vi "梦幻城堡C6~20通信.vi"() -> ()   [LabVIEW 2016, in "环境动力监测库.lvlib" / "UPS库.lvlib"]
uses:
  <vilib>/Instr/_visa.llb/VISA Configure Serial Port (Instr).vi
panel:
  out "Status-WA":T1
  out "Status-Q6":T2
  in  "open":bool
  in  "close":bool
  out "通信指示":bool
  in  "关机":bool
  in  "功率查询":bool
  in  "状态查询":bool
  out "读取缓冲区":string
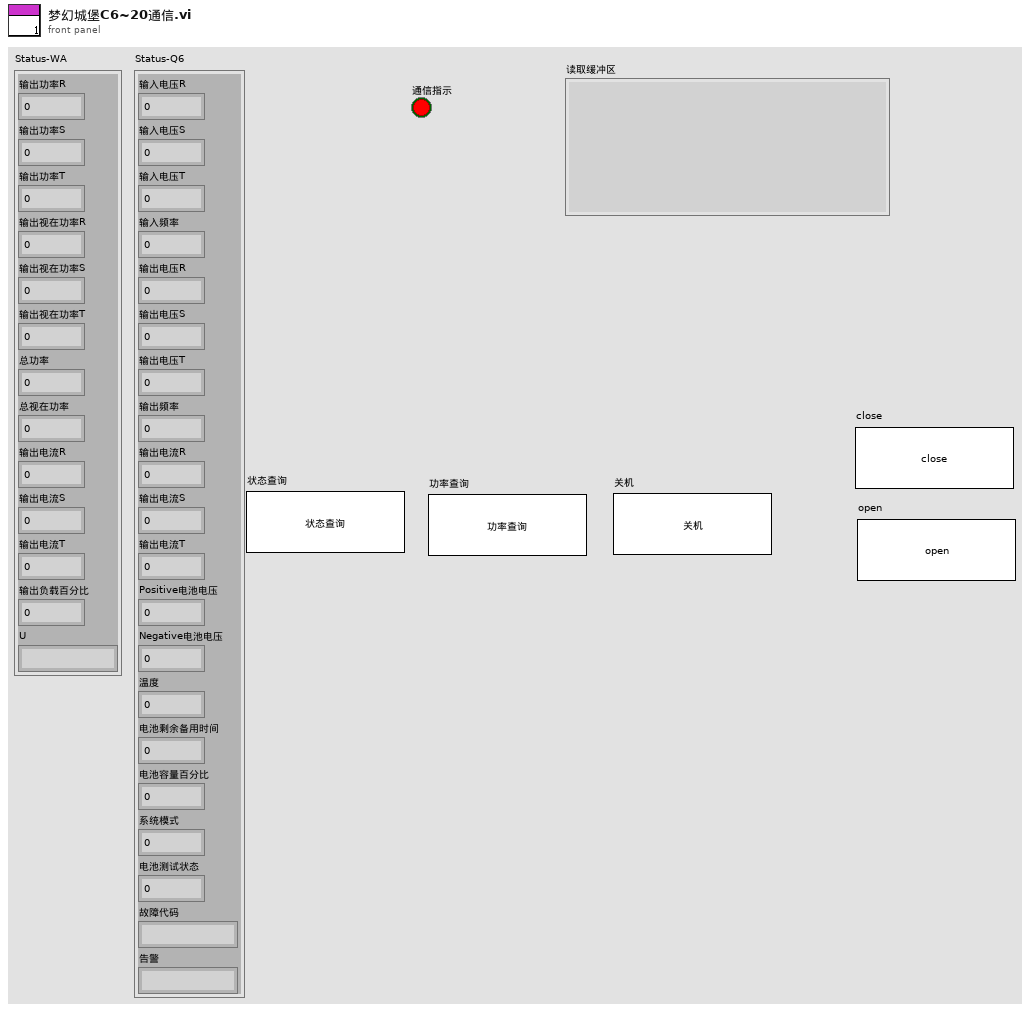
[diagram p1: front panel]
types:
  T1 = cluster{"输出功率R":dbl, "输出功率S":dbl, "输出功率T":dbl, "输出视在功率R":dbl, "输出视在功率S":dbl, "输出视在功率T":dbl, "总功率":dbl, "总视在功率":dbl, "输出电流R":dbl, "输出电流S":dbl, "输出电流T":dbl, "输出负载百分比":dbl, "U":string}
  T2 = cluster{"输入电压R":dbl, "输入电压S":dbl, "输入电压T":dbl, "输入频率":dbl, "输出电压R":dbl, "输出电压S":dbl, "输出电压T":dbl, "输出频率":dbl, "输出电流R":dbl, "输出电流S":dbl, "输出电流T":dbl, "Positive电池电压":dbl, "Negative电池电压":dbl, "温度":dbl, "电池剩余备用时间":dbl, "电池容量百分比":dbl, "系统模式":dbl, "电池测试状态":dbl, "故障代码":string, "告警":string}
  T3 = cluster{"枚举":enum16{"open", "read", "write", "close"}, "写入缓冲区":string}
  T4 = cluster{"VISA resource name":refnum<visa-resource-name>, "Serial Config":cluster{"baud rate (9600)":u32, "stop bits (10: 1 bit)":u16, "parity (0:none)":enum16{"None", "Odd", "Even", "Mark", "Space"}, "data bits (8)":u16, "timeout (10sec)":u32}, "型号选择":enum16{"山特UPSC1~3", "山特UPSC6~20", "华为UPS2000-G-(1-3KVA)"}, "HW-UPS-2000 MB session":refnum<class "MB_Master.lvclass">, "连接方式":enum16{"串口", "TCP"}, "IP":string, "Port":string}
  T5 = cluster{"baud rate (9600)":u32, "stop bits (10: 1 bit)":u16, "parity (0:none)":enum16{"None", "Odd", "Even", "Mark", "Space"}, "data bits (8)":u16, "timeout (10sec)":u32}
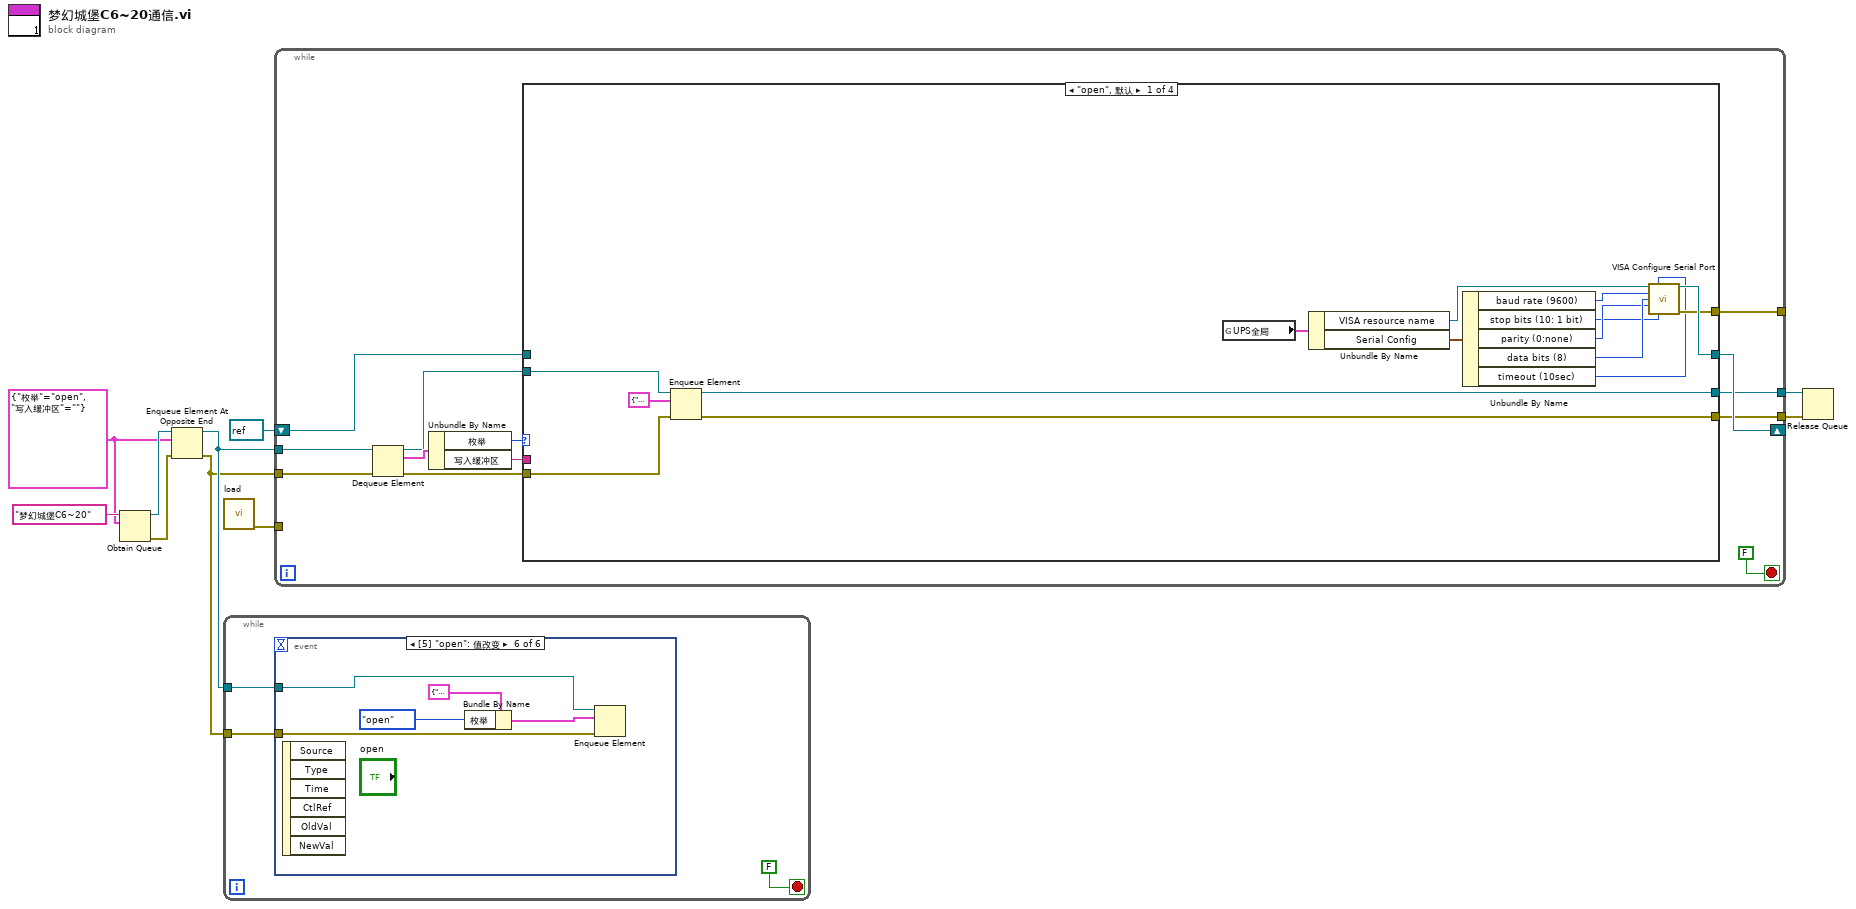
[diagram p0: block diagram]
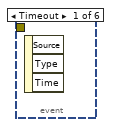
[diagram p2: hidden frame]
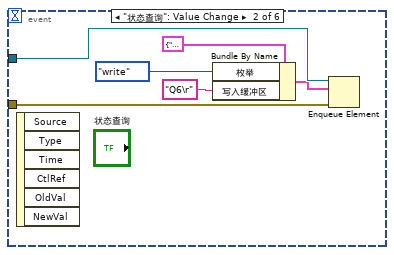
[diagram p3: hidden frame]
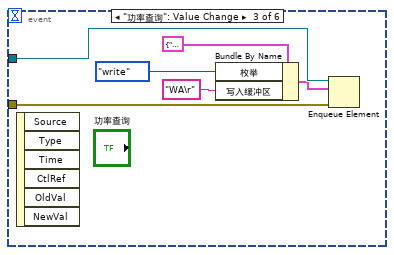
[diagram p4: hidden frame]
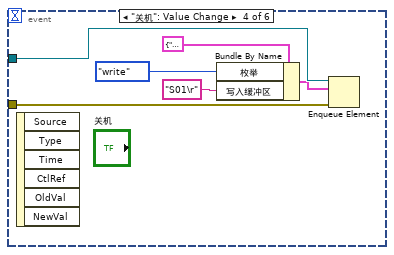
[diagram p5: hidden frame]
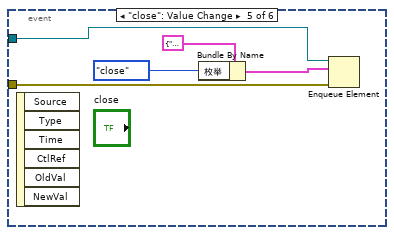
[diagram p6: hidden frame]
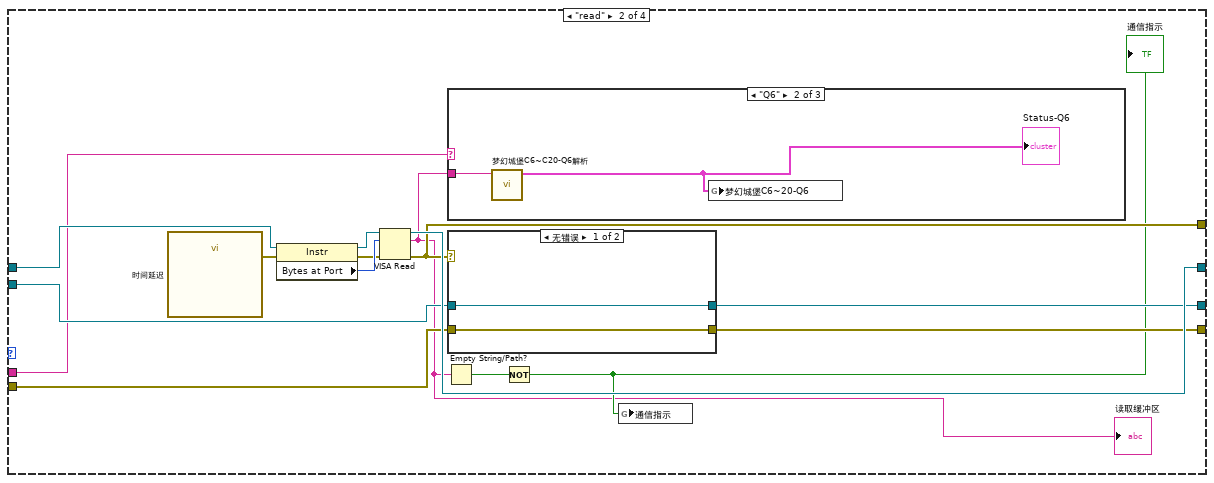
[diagram p7: hidden frame]
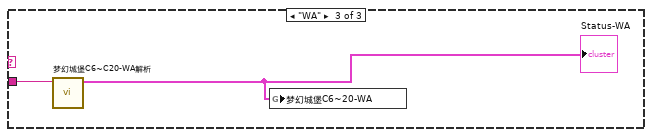
[diagram p9: hidden frame]
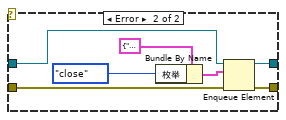
[diagram p10: hidden frame]
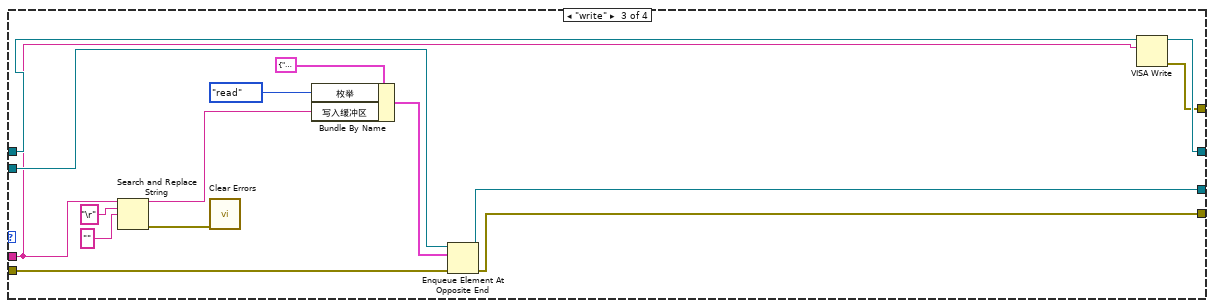
[diagram p11: hidden frame]
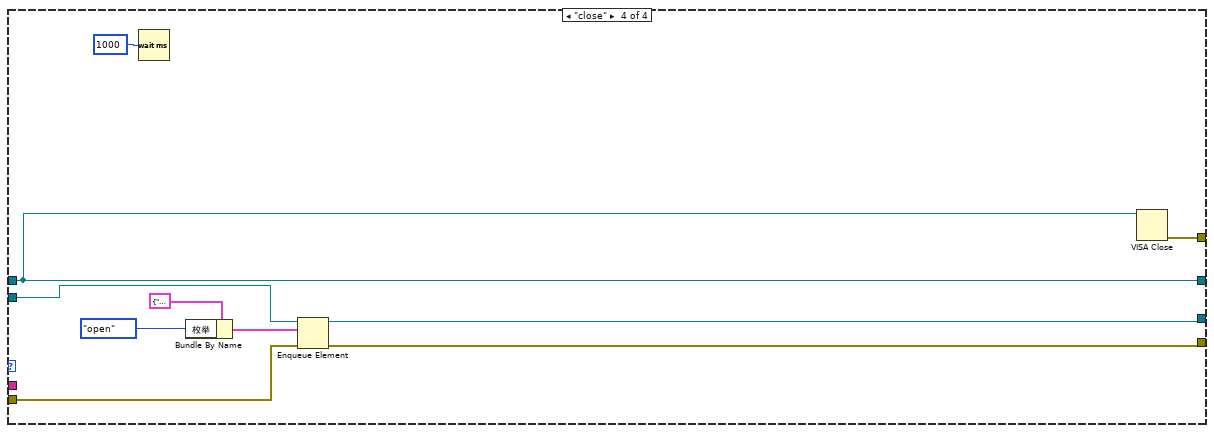
[diagram p12: hidden frame]
diagram:
  w5 = T3 {"枚举"=enum."open", "写入缓冲区"=""}
  n1 = Obtain Queue(name (unnamed)="梦幻城堡C6~20" ("名称（未命名）"), element data type=w5) -> (queue out=w9:refnum<queue>, error out=w8:errorcluster)  [unwired: 3 in, 1 out]
  n2 = Enqueue Element At Opposite End(queue=w9, element=w5, error in (no error)=w8) -> (queue out=w7:refnum<queue>, error out=w6:errorcluster)  [unwired: 1 in, 1 out]
  n3 = call "load.vi"() -> ("error out"=w1:errorcluster)  [unwired: 11 in]
  n4 = while {
    tunnel: w7 -> [w12]
    tunnel: w6 -> [w11]
    stop <- FALSE stop-if-true
    n5 = event shown="[5] \"open\": 值改变" {
      selector: _ -> [_ _ _ _ _ _]
      dyn-events: _ -> [_ _ _ _ _ _]
      timeout: _ -> [_ _ _ _ _ _]
      tunnel: w12 -> [_ w19 w25 w31 w36 w41]
      tunnel: w11 -> [_ w18 w24 w30 w35 w40]
      event Timeout {
        n6 = event-data() -> ()  [unwired: 1 in, 3 out]
      }
      event "状态查询": Value Change {
        n7 = event-data() -> ()  [unwired: 1 in, 6 out]
        n8 = Bundle By Name(cluster=T3 {"枚举"=enum."open", "写入缓冲区"=""}, "枚举"=enum16{"open", "read", "write", "close"}."write" ("元素"), "写入缓冲区"="Q6\r") -> (w14:T3)
        n9 = Enqueue Element(queue=w19, element=w14, error in (no error)=w18) -> ()  [unwired: 1 in, 3 out]
      }
      event "功率查询": Value Change {
        n10 = event-data() -> ()  [unwired: 1 in, 6 out]
        n11 = Bundle By Name(cluster=T3 {"枚举"=enum."open", "写入缓冲区"=""}, "枚举"=enum16{"open", "read", "write", "close"}."write" ("元素"), "写入缓冲区"="WA\r") -> (w20:T3)
        n12 = Enqueue Element(queue=w25, element=w20, error in (no error)=w24) -> ()  [unwired: 1 in, 3 out]
      }
      event "关机": Value Change {
        n13 = event-data() -> ()  [unwired: 1 in, 6 out]
        n14 = Bundle By Name(cluster=T3 {"枚举"=enum."open", "写入缓冲区"=""}, "枚举"=enum16{"open", "read", "write", "close"}."write" ("元素"), "写入缓冲区"="S01\r") -> (w26:T3)
        n15 = Enqueue Element(queue=w31, element=w26, error in (no error)=w30) -> ()  [unwired: 1 in, 3 out]
      }
      event "close": Value Change {
        n16 = event-data() -> ()  [unwired: 1 in, 6 out]
        n17 = Bundle By Name(cluster=T3 {"枚举"=enum."open", "写入缓冲区"=""}, "枚举"=enum16{"open", "read", "write", "close"}."close") -> (w32:T3)
        n18 = Enqueue Element(queue=w36, element=w32, error in (no error)=w35) -> ()  [unwired: 1 in, 3 out]
      }
      event "open": Value Change {
        n19 = event-data() -> ()  [unwired: 1 in, 6 out]
        n20 = Bundle By Name(cluster=T3 {"枚举"=enum."open", "写入缓冲区"=""}, "枚举"=enum16{"open", "read", "write", "close"}."open") -> (w37:T3)
        n21 = Enqueue Element(queue=w41, element=w37, error in (no error)=w40) -> ()  [unwired: 1 in, 3 out]
      }
    }
  }
  n22 = while {
    shift-right: [w54] -> _
    shift-left: refnum<visa-resource-name> refnum ("VISA resource name out") -> [w53]
    tunnel: [w52] -> _
    tunnel: w7 -> [w50]
    tunnel: w6 -> [w49]
    tunnel: [w44] -> w3
    tunnel: [w43] -> w2
    tunnel: w1 -> [_]
    stop <- FALSE stop-if-true
    n23 = Dequeue Element(queue=w50, error in (no error)=w49) -> (queue out=w46:refnum<queue>, element=w48:T3, error out=w45:errorcluster)  [unwired: 1 in, 1 out]
    n24 = Unbundle By Name(w48) -> ("枚举"=w47:enum16{"open", "read", "write", "close"}, "写入缓冲区"=w42:string)
    n25 = case shown="\"open\", 默认" w47 {
      tunnel: [w69 w81 w111 w121] -> w54
      tunnel: w53 -> [_ w84 w112 w121]
      tunnel: [w68 w79 w110 w122] -> w52
      tunnel: w46 -> [w61 w78 w103 w117]
      tunnel: w45 -> [w60 w77 w102 w116]
      tunnel: [w59 w76 w101 w115] -> w44
      tunnel: [w58 w75 w100 w114] -> w43
      tunnel: w42 -> [_ w74 w98 _]
      frame "open", Default {
        n26 = Enqueue Element(queue=w61, element=T3 {"枚举"=enum."read", "写入缓冲区"=""}, error in (no error)=w60) -> (queue out=w59:refnum<queue>, error out=w58:errorcluster)  [unwired: 1 in, 1 out]
        n27 = global read "断电保存全局变量.vi" "UPS全局"() -> (w57:T4)
        n28 = Unbundle By Name(w57) -> ("VISA resource name"=w55:refnum<visa-resource-name>, "Serial Config"=w56:T5)
        n29 = Unbundle By Name(w56) -> ("baud rate (9600)"=w66:u32, "stop bits (10: 1 bit)"=w63:u16, "parity (0:none)"=w64:enum16{"None", "Odd", "Even", "Mark", "Space"}, "data bits (8)"=w65:u16, "timeout (10sec)"=w67:u32)
        n30 = call-poly "VISA Configure Serial Port"("VISA resource name"=w55, "timeout (10sec)"=w67, "baud rate (9600)"=w66, "data bits (8)"=w65, "parity (0:none)"=w64, "stop bits (10: 1 bit)"=w63) -> ("VISA resource name out"=w69:refnum<visa-resource-name>, "error out"=w68:errorcluster)  [unwired: 8 in]
      }
      frame "read" {
        n31 = call "时间延迟"() -> ("error out"=w80:errorcluster)  [unwired: 11 in]
        n32 = property class="Instr"(reference=w84, error in=w80) -> (reference out=w82:refnum<visa-resource-name>, error out=w73:errorcluster, "Bytes at Port"=w83:u32)
        n33 = VISA Read(VISA resource name=w82, byte count=w83, error in (no error)=w73) -> (VISA resource name out=w81:refnum<visa-resource-name>, read buffer=w71:string, error out=w79:errorcluster)  [unwired: 1 out]
        "读取缓冲区" <- w71
        n34 = Empty String/Path?(string/path=w71) -> (empty?=w70:bool)
        n35 = case shown="\"Q6\"" w74 {
          tunnel: w71 -> [_ w86 w88]
          frame "假", Default {
          }
          frame "Q6" {
            n36 = call "梦幻城堡C6~C20-Q6解析.vi"("读取缓冲区"=w86) -> ("Status"=w85:T2)  [unwired: 10 in]
            "Status-Q6" <- w85
            n37 = global write "UPS内部交互全局.vi" "梦幻城堡C6~20-Q6"(w85) -> ()
          }
          frame "WA" {
            n38 = call "梦幻城堡C6~C20-WA解析.vi"("读取缓冲区"=w88) -> ("Status"=w87:T1)  [unwired: 10 in]
            "Status-WA" <- w87
            n39 = global write "UPS内部交互全局.vi" "梦幻城堡C6~20-WA"(w87) -> ()
          }
        }
        n40 = case shown="无错误" w79 {
          tunnel: w78 -> [w90 w91]
          tunnel: w77 -> [w89 w94]
          tunnel: [w90 w93] -> w76
          tunnel: [w89 w92] -> w75
          frame No Error {
          }
          frame Error {
            n41 = Bundle By Name(cluster=T3 {"枚举"=enum."open", "写入缓冲区"=""}, "枚举"=enum16{"open", "read", "write", "close"}."close") -> (w96:T3)
            n42 = Enqueue Element(queue=w91, element=w96, error in (no error)=w94) -> (queue out=w93:refnum<queue>, error out=w92:errorcluster)  [unwired: 1 in, 1 out]
          }
        }
        n43 = Not(x=w70) -> (.not. x?=w72:bool)
        "通信指示" <- w72
        n44 = global write "UPS内部交互全局.vi" "通信指示"(w72) -> ()
      }
      frame "write" {
        n45 = Search and Replace String(input string=w98, search string="\r" ("搜索字符串"), replace string="" ("替换字符串(\"\")")) -> (result string=w99:string, error out=w107:errorcluster)  [unwired: 5 in, 2 out]
        n46 = call <vilib>:"Clear Errors.vi"("error in (no error)"=w107) -> ()  [unwired: 5 in, 2 out]
        n47 = Bundle By Name(cluster=T3 {"枚举"=enum."open", "写入缓冲区"=""}, "枚举"=enum16{"open", "read", "write", "close"}."read", "写入缓冲区"=w99) -> (w104:T3)
        n48 = Enqueue Element At Opposite End(queue=w103, element=w104, error in (no error)=w102) -> (queue out=w101:refnum<queue>, error out=w100:errorcluster)  [unwired: 1 in, 1 out]
        n49 = VISA Write(VISA resource name=w112, write buffer=w98) -> (VISA resource name out=w111:refnum<visa-resource-name>, error out=w110:errorcluster)  [unwired: 1 in, 1 out]
      }
      frame "close" {
        n50 = Wait (ms)(milliseconds to wait=u32 1000 ("等待时间（毫秒）")) -> ()  [unwired: 1 out]
        n51 = Bundle By Name(cluster=T3 {"枚举"=enum."open", "写入缓冲区"=""}, "枚举"=enum16{"open", "read", "write", "close"}."open") -> (w118:T3)
        n52 = Enqueue Element(queue=w117, element=w118, error in (no error)=w116) -> (queue out=w115:refnum<queue>, error out=w114:errorcluster)  [unwired: 1 in, 1 out]
        n53 = VISA Close(VISA resource name=w121) -> (error out=w122:errorcluster)  [unwired: 1 in]
      }
    }
  }
  n54 = Release Queue(queue=w3, error in (no error)=w2) -> ()  [unwired: 1 in, 3 out]
